vi "CreateDirectoryIfNonexistent.vi"(11 "selected path":path) -> (3 "path":path)   [LabVIEW 2016]
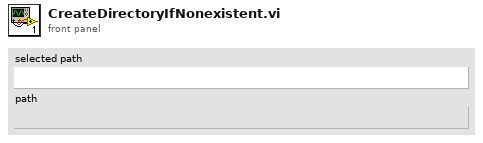
[diagram p1: front panel]
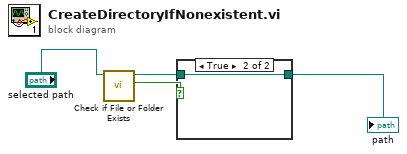
[diagram p0: block diagram]
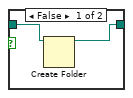
[diagram p2: hidden frame]
diagram:
  n1 = call <vilib>:"Check if File or Folder Exists.vi"("path"="selected path") -> ("file or folder exists?"=w3:bool, "dup path"=w2:path)  [unwired: 8 in, 1 out]
  n2 = case shown="True" w3 {
    tunnel: w2 -> [w6 w7]
    tunnel: [w5 w7] -> w1
    frame False {
      n3 = Create Folder(path (use dialog)=w6) -> (created path=w5:path)  [unwired: 2 in, 2 out]
    }
    frame True {
    }
  }
  "path" <- w1
